vi "减计数器.vi"(8 "error in":errorcluster, 9 "preset value":u32=10, 10 "load":bool, 11 "count down":bool) -> (0 "error out":errorcluster, 1 "counter value":u32, 3 "done":bool)   [LabVIEW 2012]
uses:
  <vilib>/ptbypt/NI_PtbyPt.lvlib
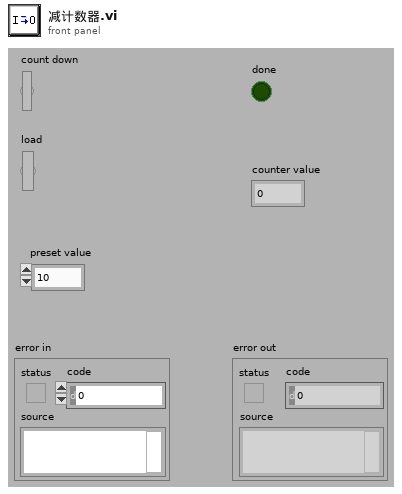
[diagram p1: front panel]
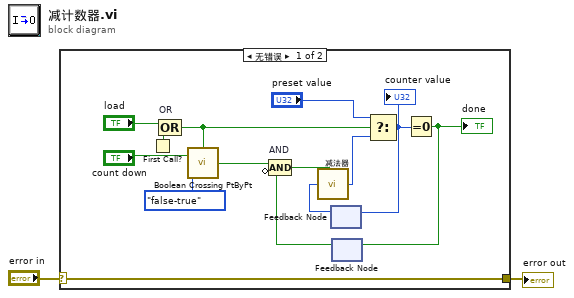
[diagram p0: block diagram]
diagram:
  n1 = case shown="无错误" "error in" {
    selector: "error in" -> [w16 w17]
    tunnel: [w16 w17] -> w2
    frame No Error {
      n2 = First Call?() -> (First Call?: T/F=w12:bool)
      n3 = Compound Arithmetic op=OR "OR"("load", w12) -> (w9:bool)
      n4 = call <vilib>:"Boolean Crossing PtByPt.vi"("initialize"=w9, "direction"=enum16{"either", "false-true", "true-false"}."false-true", "input"="count down") -> ("crossing"=w7:bool)
      n5 = feedback #1() -> (w4:u32)  [unwired: 1 in]
      n6 = feedback #2() -> (w6:bool)  [unwired: 1 in]
      n7 = Compound Arithmetic op=AND "AND"(w7, invert w6) -> (w5:bool)
      n8 = call-poly "减法器.vi"("Enable(T)"=w5, "In"=w4) -> ("Out"=w3:u32)  [unwired: 5 in]
      n9 = Select(t="preset value", s=w9, f=w3) -> (s? t:f=w8:u32)
      "counter value" <- w8
      n10 = feedback-in #1(w8) -> ()
      n11 = Equal To 0?(x=w8) -> (x = 0?=w11:bool)
      "done" <- w11
      n12 = feedback-in #2(w11) -> ()
    }
    frame Error {
    }
  }
  "error out" <- w2
